vi "Setup and Force DCPower Current for ELOAD.vi"(7 "Channel Groups?":bool, 8 "error in":errorcluster, 9 "Parameters":T1={"Supply"=0.0, "Limit"=0.0, "Aperture Time"=0.0, "Settling Time"=0.0, "Sense"=1008, "Transient Response"=1041} {"Transient Response" items=["Slow"=1041, "Normal"=1038, "Fast"=1039, "Custom"=1042]; "Sense" items=["Local"=1008, "Remote"=1009]}, 10 "Channel List":string, 11 "DCPower Handle In":refnum<k15>) -> (0 "error out":errorcluster, 3 "DCPower Handle Out":refnum<k15>)   [LabVIEW 2021, in "PMIC Common.lvlib"]
uses:
  PMIC Common.lvlib
  DCPower Parameters.ctl
  <instrlib>/niDCPower/nidcpower.llb/niDCPower Output Function.ctl
  <instrlib>/niDCPower/nidcpower.llb/niDCPower Source Mode.ctl
  <instrlib>/niDCPower/nidcpower.llb/niDCPower Wait For Event - Event.ctl
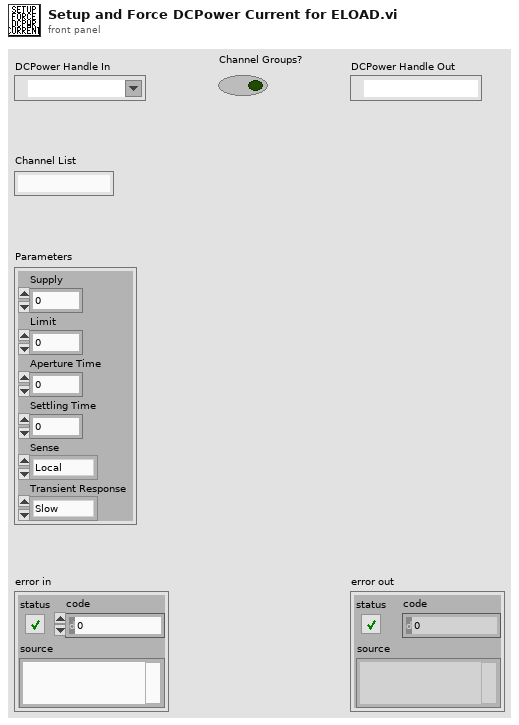
[diagram p1: front panel]
types:
  T1 = typedef "PMIC Common.lvlib/DCPower Parameters.ctl" = cluster{"Supply":dbl, "Limit":dbl, "Aperture Time":dbl, "Settling Time":dbl, "Sense":i32, "Transient Response":i32}
  T2 = typedef "niDCPower Wait For Event - Event.ctl" = i32
  T3 = typedef "niDCPower Source Mode.ctl" = i32
  T4 = typedef "niDCPower Output Function.ctl" = i32
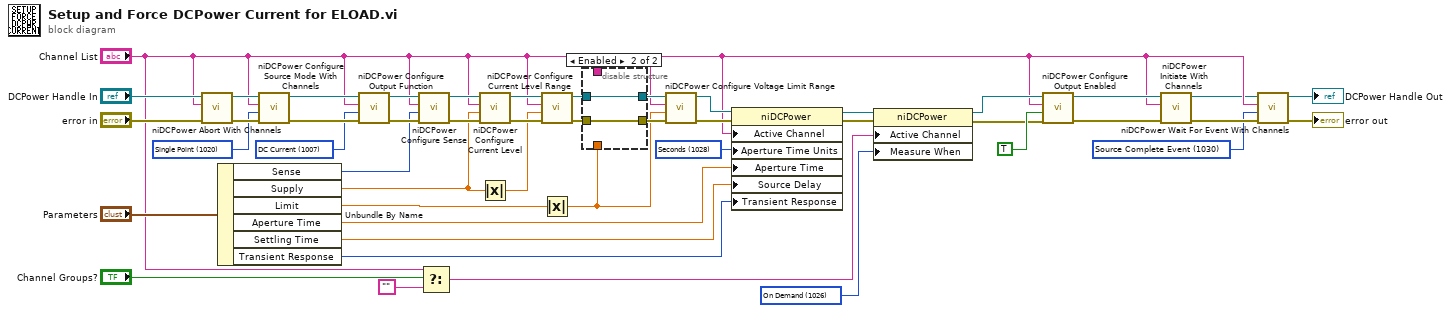
[diagram p0: block diagram]
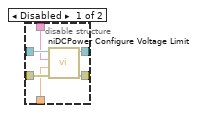
[diagram p2: hidden frame]
diagram:
  w1 = T2 1030 items=["Source Complete Event"=1030, "Measure Complete Event"=1031, "Sequence Iteration Complete Event"=1032, "Sequence Engine Done Event"=1033, "Pulse Complete Event"=1051, "Ready For Pulse Trigger Event"=1052] ("event")
  w18 = 1026 items=["Automatically after Source Complete"=1025, "On Demand"=1026, "On Measure Trigger"=1027] ("Measurement:Advanced:Measure When")
  w34 = T3 1020 items=["Single Point"=1020, "Sequence"=1021] ("source mode")
  w38 = 1028 items=["Seconds"=1028, "Power Line Cycles"=1029] ("Measurement:Aperture Time Units")
  w4 = T4 1007 items=["DC Voltage"=1006, "DC Current"=1007, "Pulse Voltage"=1049, "Pulse Current"=1050] ("output function")
  n1 = call <instrlib>:"niDCPower Abort With Channels.vi"("error in (no error)"="error in", "channel name"="Channel List", "instrument handle"="DCPower Handle In") -> ("error out"=w36:errorcluster, "instrument handle out"=w47:refnum<k15>)  [unwired: 7 in]
  n2 = Unbundle By Name("Parameters") -> ("Sense"=w11:i32, "Supply"=w10:dbl, "Limit"=w9:dbl, "Aperture Time"=w8:dbl, "Settling Time"=w7:dbl, "Transient Response"=w6:i32)
  n3 = call <instrlib>:"niDCPower Configure Source Mode With Channels.vi"("error in (no error)"=w36, "source mode"=w34, "channel name"="Channel List", "instrument handle"=w47) -> ("error out"=w35:errorcluster, "instrument handle out"=w37:refnum<k15>)  [unwired: 6 in]
  n4 = call <instrlib>:"niDCPower Configure Output Function.vi"("error in (no error)"=w35, "output function"=w4, "channel name"="Channel List", "instrument handle"=w37) -> ("error out"=w29:errorcluster, "instrument handle out"=w28:refnum<k15>)  [unwired: 6 in]
  n5 = call <instrlib>:"niDCPower Configure Sense.vi"("error in (no error)"=w29, "sense"=w11, "channel name"="Channel List", "instrument handle"=w28) -> ("error out"=w26:errorcluster, "instrument handle out"=w27:refnum<k15>)  [unwired: 6 in]
  n6 = Select(t="Channel List", s="Channel Groups?", f="") -> (s? t:f=w19:string)
  n7 = call <instrlib>:"niDCPower Configure Current Level.vi"("error in (no error)"=w26, "current level"=w10, "channel name"="Channel List", "instrument handle"=w27) -> ("error out"=w46:errorcluster, "instrument handle out"=w45:refnum<k15>)  [unwired: 6 in]
  n8 = Absolute Value(x=w10) -> (abs(x)=w25:dbl)
  n9 = call <instrlib>:"niDCPower Configure Current Level Range.vi"("error in (no error)"=w46, "current level range"=w25, "channel name"="Channel List", "instrument handle"=w45) -> ("error out"=w42:errorcluster, "instrument handle out"=w41:refnum<k15>)  [unwired: 6 in]
  n10 = Absolute Value(x=w9) -> (abs(x)=w30:dbl)
  n11 = disable-structure shown="Enabled" {
    disable-tunnel: [w53 w54] -> w44
    disable-tunnel: [w52 w55] -> w43
    disable-tunnel: w42 -> [w51 w54]
    disable-tunnel: w41 -> [w50 w55]
    disable-tunnel: w30 -> [w49 _]
    disable-tunnel: "Channel List" -> [w48 _]
    frame Disabled {
      n12 = call <instrlib>:"niDCPower Configure Voltage Limit.vi"("error in (no error)"=w51, "voltage limit"=w49, "channel name"=w48, "instrument handle"=w50) -> ("error out"=w53:errorcluster, "instrument handle out"=w52:refnum<k15>)  [unwired: 6 in]
    }
    frame Enabled {
    }
  }
  n13 = call <instrlib>:"niDCPower Configure Voltage Limit Range.vi"("error in (no error)"=w44, "voltage limit range"=w30, "channel name"="Channel List", "instrument handle"=w43) -> ("error out"=w39:errorcluster, "instrument handle out"=w40:refnum<k15>)  [unwired: 6 in]
  n14 = property class="niDCPower"(reference=w40, error in=w39, "Active Channel"="Channel List", "Aperture Time Units"=w38, "Aperture Time"=w8, "Source Delay"=w7, "Transient Response"=w6) -> (reference out=w22:refnum<k15>, error out=w24:errorcluster)
  n15 = property class="niDCPower"(reference=w22, error in=w24, "Active Channel"=w19, "Measure When"=w18) -> (reference out=w23:refnum<k15>, error out=w21:errorcluster)
  n16 = call <instrlib>:"niDCPower Configure Output Enabled.vi"("error in (no error)"=w21, "output enabled"=TRUE, "channel name"="Channel List", "instrument handle"=w23) -> ("error out"=w33:errorcluster, "instrument handle out"=w32:refnum<k15>)  [unwired: 6 in]
  n17 = call <instrlib>:"niDCPower Initiate With Channels.vi"("error in (no error)"=w33, "channel name"="Channel List", "instrument handle"=w32) -> ("error out"=w2:errorcluster, "instrument handle out"=w3:refnum<k15>)  [unwired: 7 in]
  n18 = call <instrlib>:"niDCPower Wait For Event With Channels.vi"("error in (no error)"=w2, "event"=w1, "channel name"="Channel List", "instrument handle"=w3) -> ("error out"=→"error out":errorcluster, "instrument handle out"=→"DCPower Handle Out":refnum<k15>)  [unwired: 6 in]
